vi "Open VI Clone Reference__ogtk.vi"(6 "password (\"\")":string, 8 "error in (no error)":errorcluster, 10 "vi path":path, 11 "application reference (local)":refnum<vi>) -> (0 "error out":errorcluster, 3 "clone vi reference":refnum<vi>)   [LabVIEW 2009]
doc: "This VI clones a specified VI, creates a reference to the clone by saving a copy of the VI as a VI Template and then opening a reference to the template. It then deletes the template on disk, while leaving the clone in memory. As is, this VI can only produce non-strict references to VIs. The \"type specifier VI Refnum\" should be added if you wish to \"Call by Reference\". It is suggested that you make a copy of this VI and add the type specifier for each strict reference you require. A Polymorphic VI implimentation is not realistically capable of including all possible permutations of connector panel types, which is required for strict references and used by the \"Call By Reference Node\"."
panel:
  # "Open VI Clone Reference.vi\n\nCreates a clone of a vi and returns its reference\n\nPlease visit http://www.OpenG.org to learn about the\nOpen Source LabVIEW software movement.\n\nNOTICE -- YOU MUST LEAVE THIS NOTICE IN PLACE.  PER THE TERMS OF THE LICENSE BELOW, YOU MAY SUBLICENSE THIS SOFTWARE \nIN ANY WAY THAT DOES NOT CONFLICT WITH THIS LICENSE.\n\n### BSD License (http://www.opensource.org/licenses/bsd-license.php) Begin ###\n \nCopyright (c) 2002, Jim Kring <jim@jimkring.com>\n\nAll rights reserved.\n\nRedistribution and use in source and binary forms, with or without modification, are permitted provided that the following conditions are met:\n\n    * Redistributions of source code must retain the above copyright notice, this list of conditions and the following disclaimer.\n    * Redistributions in binary form must reproduce the above copyright notice, this list of conditions and the following disclaimer in the \n       documentation and/or other materials provided with the distribution.\n    * Neither the name of SciWare, James Kring, Inc., nor the names of its contributors may be used to endorse or promote products derived \n       from this software without specific prior written permission.\n\nTHIS SOFTWARE IS PROVIDED BY THE COPYRIGHT HOLDERS AND CONTRIBUTORS \"AS IS\" AND ANY EXPRESS OR IMPLIED WARRANTIES, \nINCLUDING, BUT NOT LIMITED TO, THE IMPLIED WARRANTIES OF MERCHANTABILITY AND FITNESS FOR A PARTICULAR PURPOSE ARE \nDISCLAIMED. IN NO EVENT SHALL THE COPYRIGHT OWNER OR CONTRIBUTORS BE LIABLE FOR ANY DIRECT, INDIRECT, INCIDENTAL,\n SPECIAL, EXEMPLARY, OR CONSEQUENTIAL DAMAGES (INCLUDING, BUT NOT LIMITED TO, PROCUREMENT OF SUBSTITUTE GOODS OR \nSERVICES; LOSS OF USE, DATA, OR PROFITS; OR BUSINESS INTERRUPTION) HOWEVER CAUSED AND ON ANY THEORY OF LIABILITY, \nWHETHER IN CONTRACT, STRICT LIABILITY, OR TORT (INCLUDING NEGLIGENCE OR OTHERWISE) ARISING IN ANY WAY OUT OF THE USE \nOF THIS SOFTWARE, EVEN IF ADVISED OF THE POSSIBILITY OF SUCH DAMAGE.\n\n### BSD License End ###"
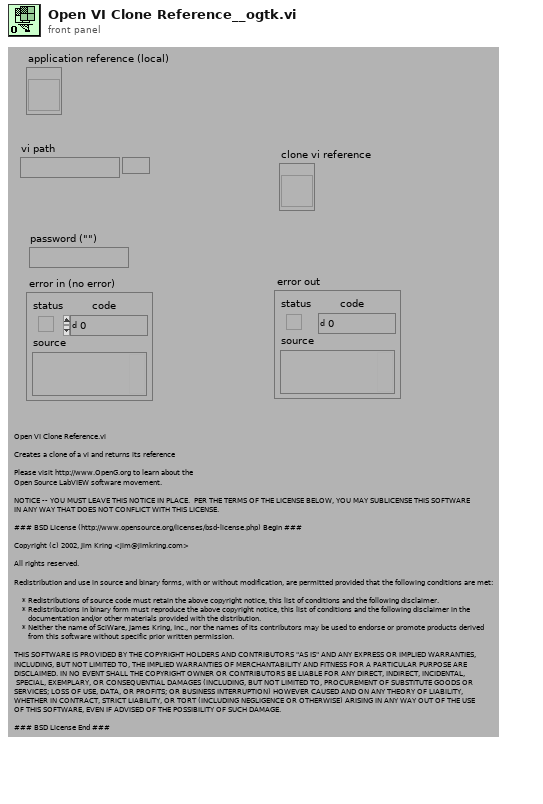
[diagram p1: front panel]
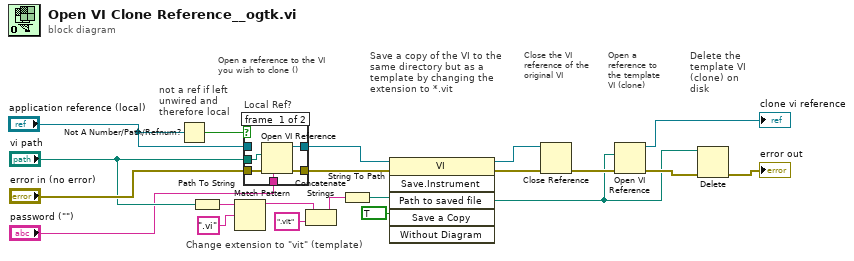
[diagram p0: block diagram]
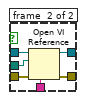
[diagram p2: hidden frame]
diagram:
  # "Change extension to \"vit\" (template)"
  # "not a ref if left unwired and therefore local"
  # "Delete the template VI (clone) on disk"
  # "Open a reference to the template VI (clone)"
  # "Close the VI reference of the original VI"
  # "Save a copy of the VI to the same directory but as a template by changing the extension to *.vit"
  # "Open a reference to the VI you wish to clone ()"
  n1 = Not A Number/Path/Refnum?(number/path/refnum="application reference (local)") -> (NaN/Path/Refnum?=w7:bool)
  n2 = Path To String(path="vi path") -> (string=w18:string)
  n3 = Match Pattern(string=w18, regular expression=".vi") -> (before substring=w17:string)  [unwired: 1 in, 3 out]
  n4 = case "Local Ref?" shown="False" w7 {
    tunnel: "vi path" -> [w25 w31]
    tunnel: [w24 w30] -> w2
    tunnel: "application reference (local)" -> [_ w27]
    tunnel: [w23 w29] -> w3
    tunnel: "error in (no error)" -> [w22 w28]
    tunnel: "password (\"\")" -> [w21 w26]
    frame #0 {
      n5 = Open VI Reference(vi path=w25, password ("")=w21, error in (no error)=w22) -> (vi reference=w23:refnum<vi>, error out=w24:errorcluster)  [unwired: 3 in]
    }
    frame #1 {
      n6 = Open VI Reference(application reference (local)=w27, vi path=w31, password ("")=w26, error in (no error)=w28) -> (vi reference=w29:refnum<vi>, error out=w30:errorcluster)  [unwired: 2 in]
    }
  }
  n7 = Concatenate Strings(w17, ".vit" ("regular expression")) -> (w15:string)
  n8 = String To Path(string=w15) -> (path=w10:path)
  n9 = invoke class="VI" method="Save.Instrument"(reference=w3, error in=w2, "Path to saved file"=w10, "Save a Copy"=TRUE) -> (reference out=w14:refnum<vi>, error out=w13:errorcluster)  [unwired: 2 in, 4 out]
  n10 = Close Reference(reference=w14, error in (no error)=w13) -> (error out=w12:errorcluster)
  n11 = Open VI Reference(vi path=w10, error in (no error)=w12) -> (vi reference=→"clone vi reference":refnum<vi>, error out=w11:errorcluster)  [unwired: 4 in]
  n12 = Delete(path (use dialog)=w10, error in=w11) -> (error out=→"error out":errorcluster)  [unwired: 3 in, 2 out]
